vi "Configure 3 mA Chan.vi"(8 "error In":errorcluster, 11 "VISA resource name in":refnum<visa-resource-name>) -> (0 "error out":errorcluster, 3 "VISA resource name out":refnum<visa-resource-name>)   [LabVIEW 2010]
uses:
  FFT_DAS/Drivers/Agilent U2722A/U2722 LabVIEW Instr Driver and Examples/Public/Configure/Configure Channel (Current).vi
  FFT_DAS/Drivers/Agilent U2722A/U2722 LabVIEW Instr Driver and Examples/Agilent U2722.lvlib
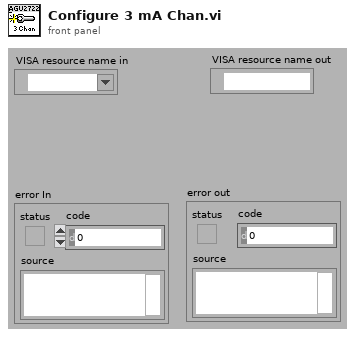
[diagram p1: front panel]
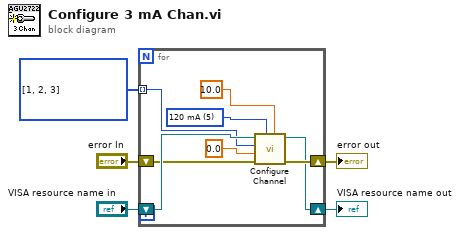
[diagram p0: block diagram]
diagram:
  w2 = u16[] [1, 2, 3] items=["Channel 1"=1, "Channel 2"=2, "Channel 3"=3] ("Array")
  n1 = for {
    tunnel: w2 -> [w12] mode=indexing
    shift-right: [w10] -> w5
    shift-left: "error In" -> [w11]
    shift-right: [w8] -> w1
    shift-left: "VISA resource name in" -> [w13]
    w9 = u16 5 items=["1 uA", "10 uA", "100 uA", "1 mA", "10 mA", "120 mA"] ("Current Range (0: 1 uA)")
    n2 = call-poly "Configure Channel.vi"("Voltage Limit (2.0 V)"=10.0, "Current Range (0: 1 uA)"=w9, "error in (no error)"=w11, "Output Level (1.0 mA)"=0.0, "Channel (1: Channel 1)"=w12, "VISA resource name"=w13) -> ("error out"=w10:errorcluster, "VISA resource name out"=w8:refnum<visa-resource-name>)  [unwired: 4 in]
  }
  "error out" <- w5
  "VISA resource name out" <- w1
